vi "Run Test.vi"(8 "error in (no error)":errorcluster, 11 "Test Template in":refnum<class "Curve Trace.lvclass">) -> (0 "error out":errorcluster, 1 "Positions":i32[](array[numeric]), 2 "Tests Passed":bool[](array[boolean]), 3 "Test Template out":refnum<class "Curve Trace.lvclass">, 5 "Fail Codes":string[](array[string]))   [LabVIEW 2015, in "Curve Trace.lvclass"]
uses:
  Curve Trace.lvclass
  CBTF Applications/Reliability Testing/Main/Rel Load Curve Tracer/Application/Application/Class/typedefs/Instrument Selector -- Enum.ctl
  Classes/Instruments/Temperature Device/ThorLabs TSP01/Class/ThorLabs TSP01.lvclass
  Classes/Instruments/DC Power Supply/DC Power Supply/Class/DC Power Supply.lvclass
  Test Class/Test Class.lvclass
  Classes/Application/Class/Application.lvclass
  CBTF Applications/Reliability Testing/Main/Rel Load Curve Tracer/Application/Application/Class/Rel Curve Tracer.lvclass
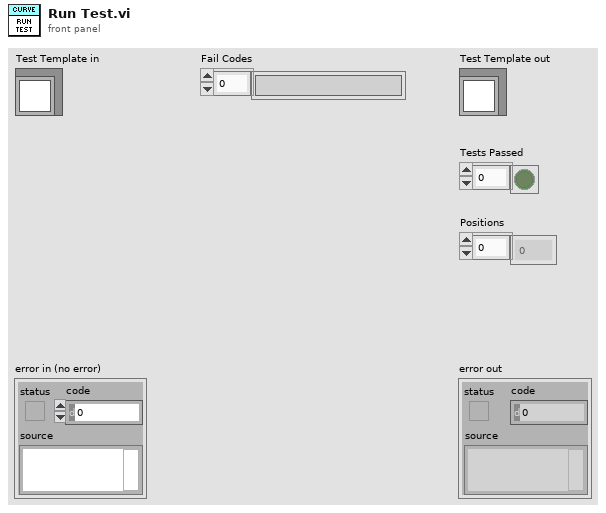
[diagram p1: front panel]
types:
  T1 = typedef "Rel Curve Tracer.lvlib/Rel Curve Tracer.lvclass/Instrument Selector -- Enum.ctl" = enum16{"DC Power Supply", "Temp Device", "Switch"}
  T2 = enum16{"Voltage RMS", "Voltage DC", "AC Current", "DC Current", "Frequency", "Real Power", "Reactive Power", "Apparent Power", "Power Factor"}
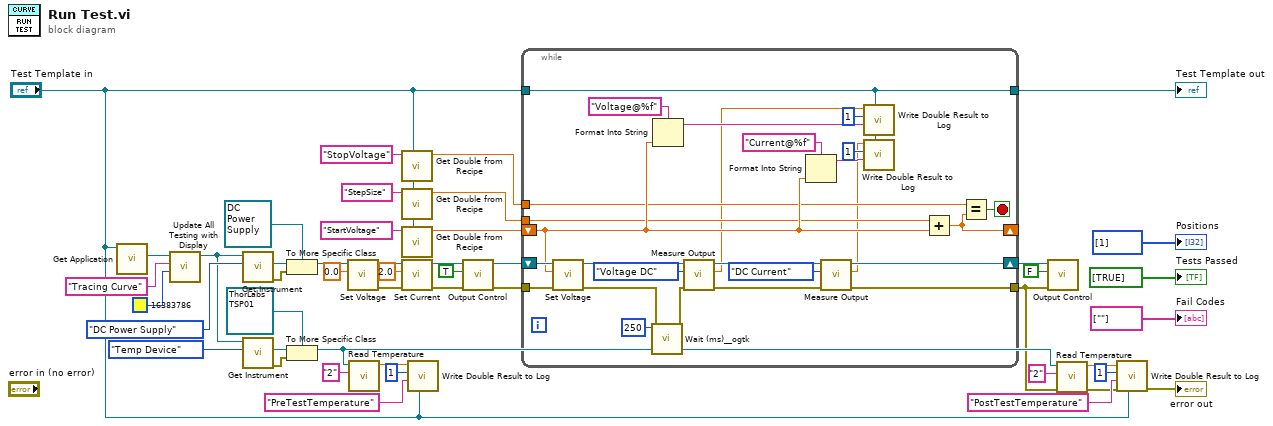
[diagram p0: block diagram]
diagram:
  n1 = call "Get Application.vi"("Test Class in"="Test Template in") -> ("Application.lvlib:Application.lvclass"=w46:refnum<class "Application.lvclass">)  [unwired: 9 in, 1 out]
  n2 = call "Update All Testing with Display.vi"("BG Color"=u32 16383786, "Message ('')"="Tracing Curve", "Application in"=w46) -> ("Application out"=w42:refnum<class "Application.lvclass">)  [unwired: 7 in, 1 out]
  n3 = call "Get Instrument.vi"("Instrument Number"=Instrument_Selector_--_Enum."DC Power Supply" ("Instrument"), "Application in"=w42) -> ("error out"=w38:errorcluster, "Instrument"=w41:refnum<class "Instrument.lvclass">)  [unwired: 7 in, 1 out]
  n4 = call "Get Instrument.vi"("Instrument Number"=Instrument_Selector_--_Enum."Temp Device" ("Instrument"), "Application in"=w42) -> ("error out"=w39:errorcluster, "Instrument"=w40:refnum<class "Instrument.lvclass">)  [unwired: 7 in, 1 out]
  n5 = To More Specific Class(target class=refnum<class "DC Power Supply.lvclass"> refnum ("DC Power Supply.lvlib:DC Power Supply.lvclass"), reference=w41, error in=w38) -> (specific class reference=w35:refnum<class "DC Power Supply.lvclass">)  [unwired: 1 out]
  n6 = To More Specific Class(target class=refnum<class "ThorLabs TSP01.lvclass"> refnum ("ThorLabs TSP01.lvlib:ThorLabs TSP01.lvclass"), reference=w40, error in=w39) -> (specific class reference=w28:refnum<class "ThorLabs TSP01.lvclass">)  [unwired: 1 out]
  n7 = call-dynamic "Set Voltage.vi"("Voltage (0.0 V)"=0.0 ("Voltage (0.0 VDC)"), "Acrobat Template in"=w35) -> ("error out"=w31:errorcluster, "Acrobat Template out"=w33:refnum<class "DC Power Supply.lvclass">)  [unwired: 8 in]
  n8 = call-dynamic "Read Temperature.vi"("Channel"="2", "Acrobat Template in"=w28) -> ("Temperature out"=w16:dbl)  [unwired: 8 in, 1 out]
  n9 = call "Get Double from Recipe.vi"("Test Class in"="Test Template in", "Name"="StopVoltage") -> ("Value"=w4:dbl)  [unwired: 7 in, 2 out]
  n10 = call "Get Double from Recipe.vi"("Test Class in"="Test Template in", "Name"="StepSize") -> ("Value"=w7:dbl)  [unwired: 7 in, 2 out]
  n11 = call "Get Double from Recipe.vi"("Test Class in"="Test Template in", "Name"="StartVoltage") -> ("Value"=w9:dbl)  [unwired: 7 in, 2 out]
  n12 = call-dynamic "Set Current.vi"("error in (no error)"=w31, "Current (0.0A)"=2.0, "Acrobat Template in"=w33) -> ("error out"=w22:errorcluster, "Acrobat Template out"=w24:refnum<class "DC Power Supply.lvclass">)  [unwired: 7 in]
  n13 = call "Write Double Result to Log.vi"("Test Class in"="Test Template in", "Label"="PreTestTemperature", "Position"=u32 1, "Value"=w16) -> ()  [unwired: 7 in, 1 out]
  n14 = call-dynamic "Output Control.vi"("error in (no error)"=w22, "Enabled"=TRUE, "Acrobat Template in"=w24) -> ("error out"=w21:errorcluster, "Acrobat Template out"=w23:refnum<class "DC Power Supply.lvclass">)  [unwired: 7 in]
  n15 = while {
    tunnel: w21 -> [w72]
    shift-right: [w62] -> _
    shift-left: w9 -> [w63]
    shift-right: [w51] -> w17
    shift-left: w23 -> [w73]
    tunnel: [w49] -> w18
    tunnel: [w66] -> w26
    tunnel: "Test Template in" -> [w66]
    tunnel: w7 -> [w61]
    tunnel: w4 -> [w60]
    stop <- w71 stop-if-true
    n16 = call-dynamic "Set Voltage.vi"("error in (no error)"=w72, "Voltage (0.0 V)"=w63, "Acrobat Template in"=w73) -> ("error out"=w59:errorcluster, "Acrobat Template out"=w57:refnum<class "DC Power Supply.lvclass">)  [unwired: 7 in]
    n17 = call <userlib>:"Wait (ms)__ogtk.vi"("error in (no error)"=w59, "milliseconds to wait"=u32 250) -> ("error out"=w56:errorcluster)  [unwired: 8 in, 1 out]
    n18 = Format Into String(format string="Voltage@%f", w63) -> (resulting string=w64:string)  [unwired: 2 in, 1 out]
    n19 = call-dynamic "Measure Output.vi"("error in (no error)"=w56, "Measurement Type (0: Voltage RMS)"=T2."Voltage DC", "Acrobat Template in"=w57) -> ("error out"=w53:errorcluster, "Measurement"=w54:dbl, "Acrobat Template out"=w55:refnum<class "DC Power Supply.lvclass">)  [unwired: 6 in]
    n20 = Format Into String(format string="Current@%f", w63) -> (resulting string=w65:string)  [unwired: 2 in, 1 out]
    n21 = call-dynamic "Measure Output.vi"("error in (no error)"=w53, "Measurement Type (0: Voltage RMS)"=T2."DC Current", "Acrobat Template in"=w55) -> ("error out"=w49:errorcluster, "Measurement"=w50:dbl, "Acrobat Template out"=w51:refnum<class "DC Power Supply.lvclass">)  [unwired: 6 in]
    n22 = call "Write Double Result to Log.vi"("Test Class in"=w66, "Label"=w64, "Position"=u32 1, "Value"=w54) -> ()  [unwired: 7 in, 1 out]
    n23 = call "Write Double Result to Log.vi"("Test Class in"=w66, "Label"=w65, "Position"=u32 1, "Value"=w50) -> ()  [unwired: 7 in, 1 out]
    n24 = Add(x=w61, y=w63) -> (x+y=w62:dbl)
    n25 = Equal?(x=w60, y=w62) -> (x = y?=w71:bool)
  }
  "Test Template out" <- w26
  n26 = call-dynamic "Output Control.vi"("error in (no error)"=w18, "Enabled"=FALSE, "Acrobat Template in"=w17) -> ()  [unwired: 7 in, 2 out]
  n27 = call-dynamic "Read Temperature.vi"("error in (no error)"=w18, "Channel"="2", "Acrobat Template in"=w28) -> ("error out"=w3:errorcluster, "Temperature out"=w11:dbl)  [unwired: 7 in]
  n28 = call "Write Double Result to Log.vi"("Test Class in"="Test Template in", "error in (no error)"=w3, "Label"="PostTestTemperature", "Position"=u32 1, "Value"=w11) -> ("error out"=→"error out":errorcluster)  [unwired: 6 in]
  "Tests Passed" <- bool[] [TRUE] ("Tests Passed")
  "Fail Codes" <- string[] [""] ("Fail Codes")
  "Positions" <- i32[] [1] ("Positions")
